vi "escribeEnTabla.vi"(8 "error in (no error)":errorcluster, 9 "parametros":string[](array[string]), 10 "col":i32=2, 11 "tabla in":string[][](array[string])) -> (0 "error out":errorcluster, 3 "tabla out":string[][](array[string]))   [LabVIEW 2019]
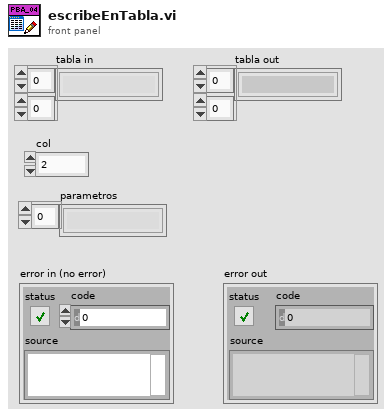
[diagram p1: front panel]
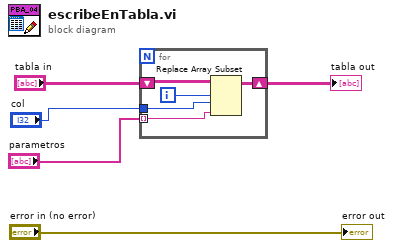
[diagram p0: block diagram]
diagram:
  n1 = for {
    shift-right: [w9] -> w5
    shift-left: "tabla in" -> [w10]
    tunnel: "parametros" -> [w7] mode=indexing
    tunnel: "col" -> [w6]
    i -> [w8]
    n2 = Replace Array Subset(array=w10, new element=w7, index (row)=w8, index (col)=w6) -> (w9:string[][])
  }
  "tabla out" <- w5
  "error out" <- "error in (no error)"
